vi "StateMachine.vi"(0 "JSONRPC Server in":refnum<class "JSONRPC Server.lvclass">, 1 "IFw session":refnum<class "niInstr FIFO Register Bus v1 Host.lvclass">, 2 "FPGA Ref":refnum<k20>, 5 "SM inputs":T2, 9 "State In":T1, 11 "error in (no error)":errorcluster) -> (4 "SM outputs":T3, 6 "State Out":T1, 15 "error out":errorcluster)   [LabVIEW 2017, in "AppStateMachine runtime.lvclass"]
uses:
  AppStateMachine runtime.lvclass
  State.ctl
  <vilib>/NI/NI JSONRPC Server Framework/Classes/Server/JSONRPC Server.lvclass
  result user data.ctl
  parameter user data.ctl
  <instrlib>/_niInstr/FIFO Register Bus/v1/Host/niInstr FIFO Register Bus v1 Host.lvclass
  FPGA/FPGAtypedef.ctl
  Support/methods.ctl
  <vilib>/NI/NI JSONRPC Server Framework/Classes/Request/Request.lvclass/Request.ctl
  Responses/ResouceUsage.ctl
  <vilib>/NI/NI JSONRPC Server Framework/Classes/Request/Read method.vi
  <vilib>/NI/NI JSONRPC Server Framework/Classes/Request/Read params.vi
  <vilib>/NI/NI JSONRPC Server Framework/Classes/Server/Add Response (Result from Request).vi
  <vilib>/LVH/i3 JSON/JSON Generation/Create Value Files/Create Value - String.vi
  <vilib>/Utility/error.llb/Error Cluster From Error Code.vi
  <vilib>/rvi/errors/niLvFpgaAdjustHostInterfaceError.vi
  <vilib>/NI/NI JSONRPC Server Framework/Classes/Request/Request.lvclass
  <vilib>/rvi/interface/nirviReadWriteControl/nirviReadWriteControl.xnode
  <vilib>/NI/NI JSONRPC Server Framework/Classes/params/params.lvclass
  <vilib>/LVH/i3 JSON/i3-json.lvlib
  NiFpgaLv.dll
  <vilib>/rvi/interface/Simulation/niFpgaSimulationCallBeginRW.vi
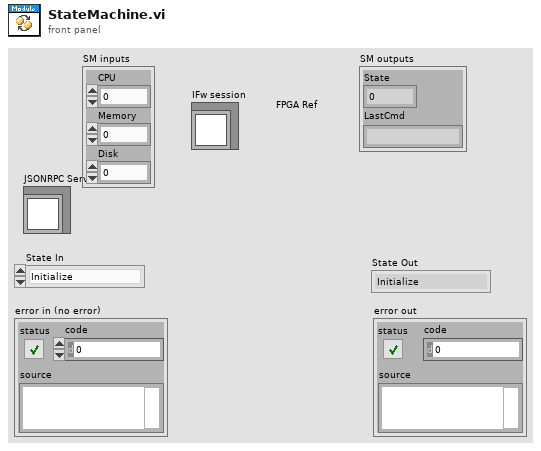
[diagram p1: front panel]
types:
  T1 = typedef "AppStateMachine runtime.lvclass/State.ctl" = enum16{"Initialize", "Idle", "Starting", "Running", "Stopping"}
  T2 = typedef "AppStateMachine runtime.lvclass/parameter user data.ctl" = cluster{"CPU":dbl, "Memory":dbl, "Disk":dbl}
  T3 = typedef "AppStateMachine runtime.lvclass/result user data.ctl" = cluster{"State":u16, "LastCmd":string}
  T4 = typedef "FPGAtypedef.ctl" = refnum<k20>
  T5 = typedef "methods.ctl" = enum16{"none", "echo", "GetResourceUsage", "CheckConnection", "GoToSafeState", "AvailableLogs", "ForceLogTrigger"}
  T6 = typedef "AppStateMachine runtime.lvclass/ResouceUsage.ctl" = cluster{"CPU":dbl, "Memory":dbl, "Disk":dbl}
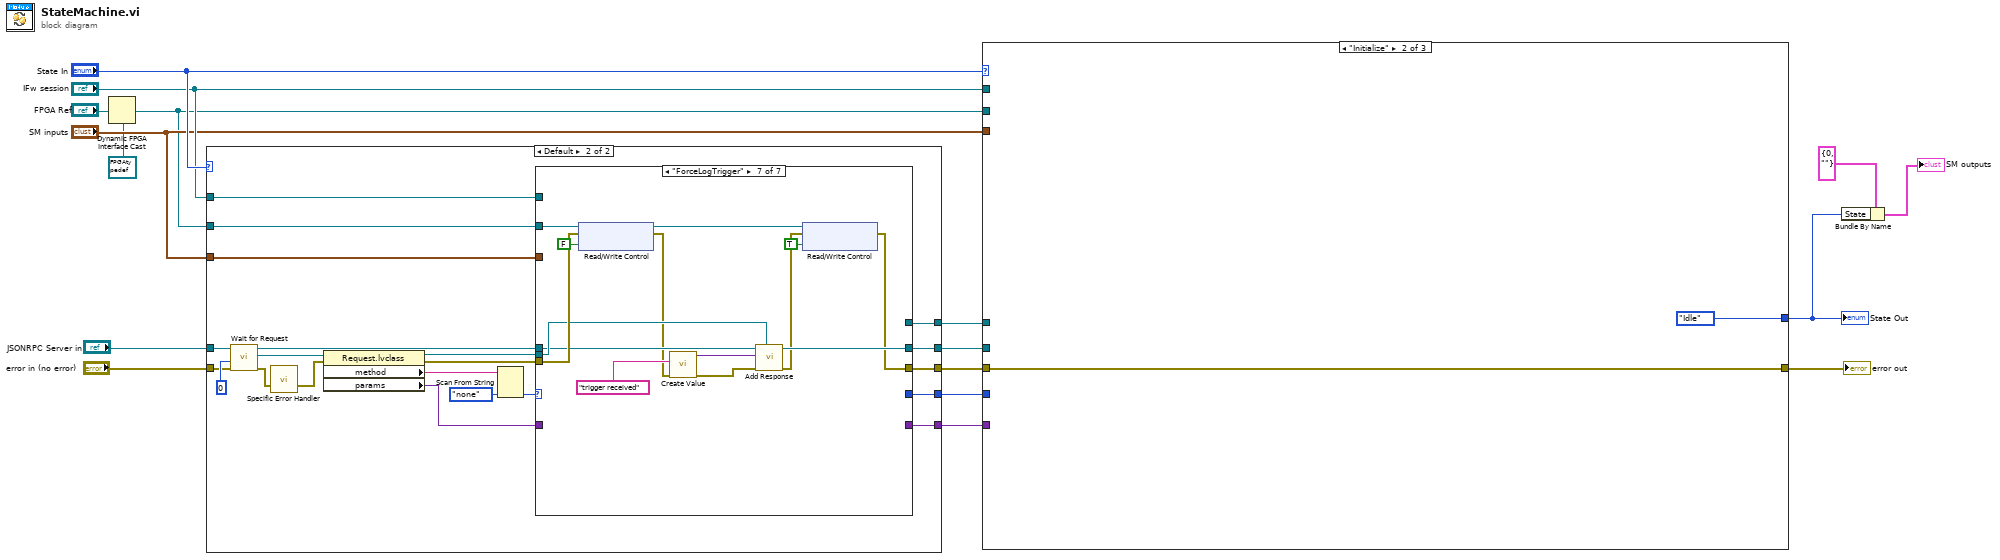
[diagram p0: block diagram]
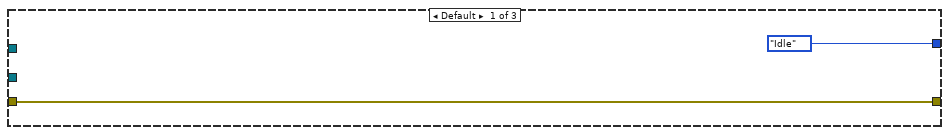
[diagram p2: hidden frame]
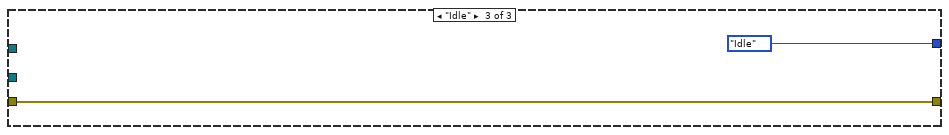
[diagram p3: hidden frame]
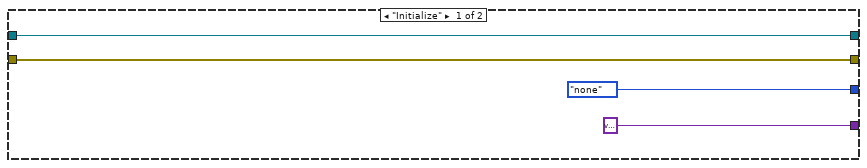
[diagram p4: hidden frame]
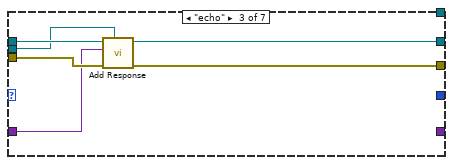
[diagram p7: hidden frame]
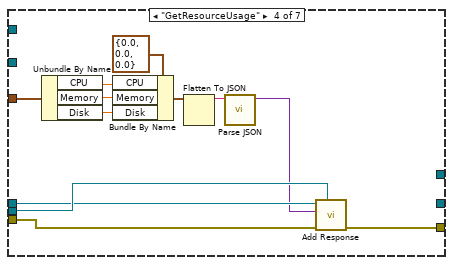
[diagram p8: hidden frame]
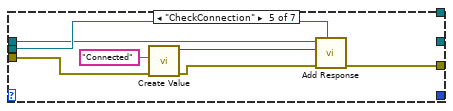
[diagram p9: hidden frame]
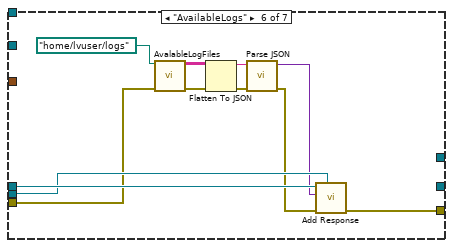
[diagram p10: hidden frame]
diagram:
  n1 = Dynamic FPGA Interface Cast(Session In=T4 refnum ("FPGA typedef"), Type="FPGA Ref") -> (Session Out=w2:T4)
  n2 = case shown="Default" "State In" {
    tunnel: "JSONRPC Server in" -> [w20 w42]
    tunnel: [_ w22] -> w17
    tunnel: "error in (no error)" -> [w21 w40]
    tunnel: [w21 w24] -> w16
    tunnel: [w20 w25] -> w9
    tunnel: [variant ("params") w23] -> w8
    tunnel: "IFw session" -> [_ w28]
    tunnel: w2 -> [_ w29]
    tunnel: [methods."none" ("methods") w27] -> w6
    tunnel: "SM inputs" -> [_ w26]
    frame "Initialize" {
    }
    frame Default {
      n3 = call <vilib>:"Wait for Request.vi"("error in (no error)"=w40, "timeout in ms (100)"=0, "Server in"=w42) -> ("error out"=w39:errorcluster, "Request"=w38:refnum<class "Request.lvclass">, "Server out"=w30:refnum<class "JSONRPC Server.lvclass">)  [unwired: 5 in, 1 out]
      n4 = call "Specific Error Handler"("Error to Check"=w39) -> ("error out"=w37:errorcluster)  [unwired: 11 in, 3 out]
      n5 = property class="Request.lvclass"(reference=w38, error in=w37) -> (reference out=w31:refnum<class "Request.lvclass">, error out=w32:errorcluster, "method"=w35:string, "params"=w33:variant)
      n6 = Scan From String(input string=w35, default 1=methods."none" ("methods")) -> (output 1=w34:T5)  [unwired: 3 in, 3 out]
      n7 = case shown="\"ForceLogTrigger\"" w34 {
        selector: w34 -> [w46 _ _ _ _ _ _]
        tunnel: w33 -> [w45 _ w47 _ _ _ _]
        tunnel: w32 -> [_ _ w49 w56 w67 w79 w95]
        tunnel: w31 -> [w43 _ w51 w55 w70 w80 w94]
        tunnel: w30 -> [w44 _ w52 w54 w69 w81 w93]
        tunnel: w29 -> [_ _ _ _ _ _ w96]
        tunnel: w28 -> [_ _ _ _ _ _ _]
        tunnel: [w46 _ _ _ _ _ _] -> w27
        tunnel: w26 -> [_ _ _ w64 _ _ _]
        tunnel: [w44 _ w50 _ _ _ w92] -> w25
        tunnel: [_ _ w48 w57 w71 w82 w83] -> w24
        tunnel: [w45 _ _ _ _ _ _] -> w23
        tunnel: [w43 _ _ _ _ _ _] -> w22
        frame Default {
        }
        frame "none" {
        }
        frame "echo" {
          n8 = call-poly <vilib>:"Add Response.vi"("Request"=w51, "error in (no error)"=w49, "Response JSON Tree In"=w47, "Server in"=w52) -> ("error out"=w48:errorcluster, "Server out"=w50:refnum<class "JSONRPC Server.lvclass">)  [unwired: 5 in, 1 out]
        }
        frame "GetResourceUsage" {
          n9 = Unbundle By Name(w64) -> ("CPU"=w60:dbl, "Memory"=w59:dbl, "Disk"=w58:dbl)
          n10 = Bundle By Name(cluster=T6 {"CPU"=0.0, "Memory"=0.0, "Disk"=0.0} ("ResourceUsage"), "CPU"=w60, "Memory"=w59, "Disk"=w58) -> (w62:T6)
          n11 = Flatten To JSON(anything=w62) -> (JSON string=w61:string)  [unwired: 2 in, 1 out]
          n12 = call <vilib>:"Parse JSON.vi"("JSON String"=w61) -> ("JSON Tree"=w53:variant)  [unwired: 7 in, 3 out]
          n13 = call-poly <vilib>:"Add Response.vi"("Request"=w55, "error in (no error)"=w56, "Response JSON Tree In"=w53, "Server in"=w54) -> ("error out"=w57:errorcluster)  [unwired: 5 in, 2 out]
        }
        frame "CheckConnection" {
          n14 = call-poly <vilib>:"Create Value.vi"("error in (no error)"=w67, "String"="Connected") -> ("error out"=w65:errorcluster, "JSON Tree"=w66:variant)  [unwired: 8 in]
          n15 = call-poly <vilib>:"Add Response.vi"("Request"=w70, "error in (no error)"=w65, "Response JSON Tree In"=w66, "Server in"=w69) -> ("error out"=w71:errorcluster)  [unwired: 5 in, 2 out]
        }
        frame "AvailableLogs" {
          n16 = call "AvalableLogFiles.vi"("path"=path "/home/lvuser/logs", "error in (no error)"=w79) -> ("FilesInfo"=w76:string[][], "error out"=w75:errorcluster)  [unwired: 12 in]
          n17 = Flatten To JSON(anything=w76, error in (no error)=w75) -> (JSON string=w77:string, 11:w74:errorcluster)  [unwired: 1 in]
          n18 = call <vilib>:"Parse JSON.vi"("error in (no error)"=w74, "JSON String"=w77) -> ("error out"=w73:errorcluster, "JSON Tree"=w72:variant)  [unwired: 6 in, 2 out]
          n19 = call-poly <vilib>:"Add Response.vi"("Request"=w80, "error in (no error)"=w73, "Response JSON Tree In"=w72, "Server in"=w81) -> ("error out"=w82:errorcluster)  [unwired: 5 in, 2 out]
        }
        frame "ForceLogTrigger" {
          n20 = xnode "Read/Write Control"("FPGA VI Reference In"=w96, "error in"=w95, "ManualTrigger"=FALSE) -> ("FPGA VI Reference Out"=w86:T4, "error out"=w89:errorcluster)
          n21 = call-poly <vilib>:"Create Value.vi"("error in (no error)"=w89, "String"="trigger received") -> ("error out"=w88:errorcluster, "JSON Tree"=w87:variant)  [unwired: 8 in]
          n22 = call-poly <vilib>:"Add Response.vi"("Request"=w94, "error in (no error)"=w88, "Response JSON Tree In"=w87, "Server in"=w93) -> ("error out"=w84:errorcluster, "Server out"=w92:refnum<class "JSONRPC Server.lvclass">)  [unwired: 5 in, 1 out]
          n23 = xnode "Read/Write Control"("FPGA VI Reference In"=w86, "error in"=w84, "ManualTrigger"=TRUE) -> ("error out"=w83:errorcluster)  [unwired: 1 out]
        }
      }
    }
  }
  n24 = case shown="\"Initialize\"" "State In" {
    tunnel: w16 -> [w97 w100 w101]
    tunnel: w17 -> [_ _ _]
    tunnel: [w97 w100 w101] -> w11
    tunnel: [State."Idle" ("State Out") State."Idle" ("State Out") State."Idle" ("State Out")] -> w10
    tunnel: w9 -> [_ _ _]
    tunnel: w8 -> [_ _ _]
    tunnel: w6 -> [_ _ _]
    tunnel: "IFw session" -> [_ _ _]
    tunnel: w2 -> [_ _ _]
    tunnel: "SM inputs" -> [_ _ _]
    frame Default {
    }
    frame "Initialize" {
    }
    frame "Idle" {
    }
  }
  "State Out" <- w10
  "error out" <- w11
  n25 = Bundle By Name(cluster=T3 {"State"=0, "LastCmd"=""} ("data cluster"), "State"=w10) -> (→"SM outputs":T3)
